vi "Channels Quiz - High Speed Streams and Tags.vi"() -> ()   [LabVIEW 2019]
doc: "After you have studied the other shipping examples to learn about channels, try this quiz to test your understanding."
uses:
  <extravilib>/ChannelInstances/High Speed Stream-i32/_Read For Replicate.vi
  <extravilib>/ChannelInstances/Tag-i32/Read With Abort.vi
  <extravilib>/ChannelInstances/Tag-i32/Write With Abort.vi
  <extravilib>/ChannelInstances/High Speed Stream-i32/Instantiate.vi
  <extravilib>/ChannelInstances/High Speed Stream-i32/)Channel.vi
  <extravilib>/ChannelInstances/High Speed Stream-i32/Abort Signal/Init Signal.vi
  <extravilib>/ChannelInstances/Tag-i32/Instantiate.vi
  <extravilib>/ChannelInstances/Tag-i32/EndpointRead.vi
  <extravilib>/ChannelInstances/Tag-i32/Endpoint.vi
  <extravilib>/ChannelInstances/High Speed Stream-i32.lvlib
  <extravilib>/ChannelInstances/Tag-i32.lvlib
panel:
  in  "Channel Type":string(combo)="High Speed Stream"
  out "element 1":i32
  in  "Stop Tag":bool
  in  "Stop Stream":bool
  out "element 0":i32
  # "Overview: Provides quiz questions related to several Channels concepts. You may wish to study the other channel examples first before attempting this quiz.\nInstructions:\n1. View the block diagram to see quiz questions related to High Speed Stream and Tag channel types.\n2. If you wish to run the VI to further understand the quiz answers, make sure you have specified the Channel Type that executes the diagram you wish to explore, and use the proper Stop button below to stop the VI."
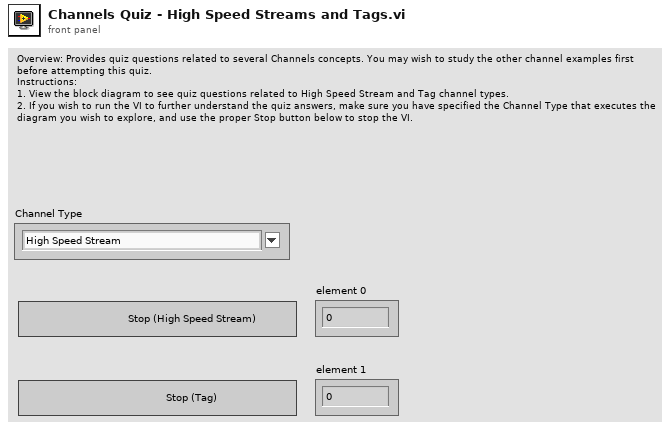
[diagram p1: front panel]
types:
  T1 = typedef "High Speed Stream-i32.lvlib/)Channel.ctl" = refnum<queue>
  T2 = typedef "Tag-i32.lvlib/))Channel.ctl" = refnum<queue>
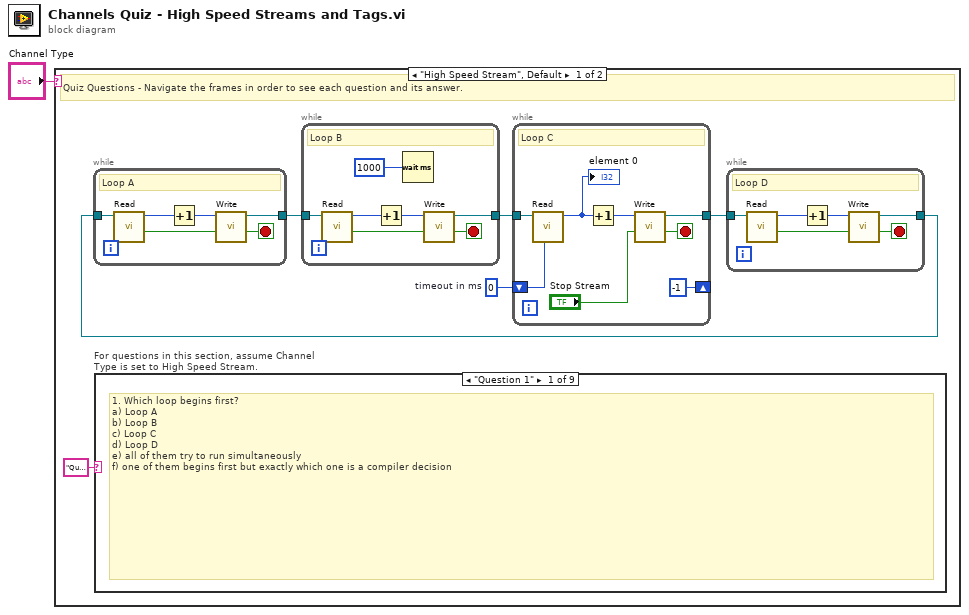
[diagram p0: block diagram]
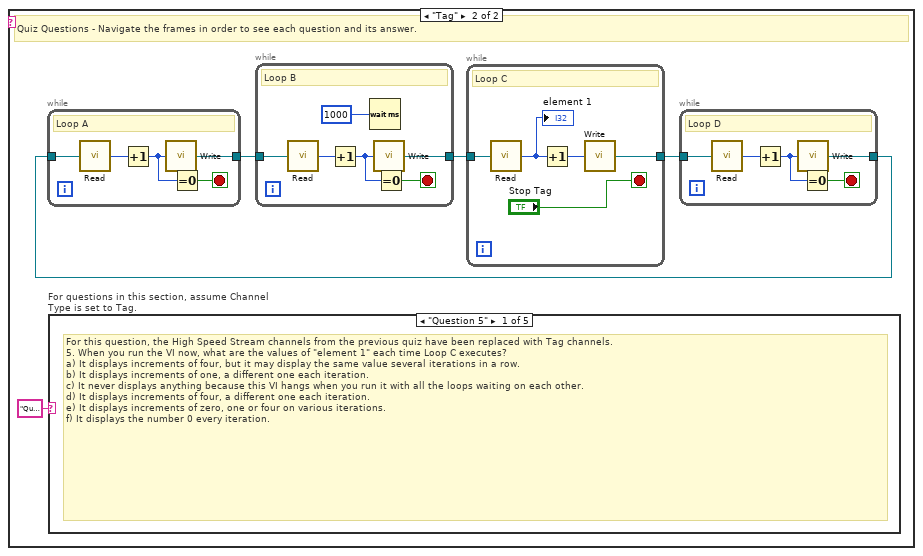
[diagram p10: hidden frame]
diagram:
  n1 = case shown="\"High Speed Stream\", Default" "Channel Type" {
    frame "High Speed Stream", Default {
      w3 = 0  # timeout in ms
      # "Quiz Questions - Navigate the frames in order to see each question and its answer."
      n2 = case "For questions in this section, assume Channel Type is set to High Speed Stream." shown="\"Question 1\"" "Question 1" {
        frame "Question 1" {
          # "1. Which loop begins first?\na) Loop A\nb) Loop B\nc) Loop C\nd) Loop D\ne) all of them try to run simultaneously\nf) one of them begins first but exactly which one is a compiler decision"
        }
        frame "Answer 1" {
          # "1. Which loop begins first?\na) Loop A\nb) Loop B\nc) Loop C\nd) Loop D\ne) all of them try to run simultaneously\nf) one of them begins first but exactly which one is a compiler decision\n\nAnswer: E. All try to begin at the same time. Channel wires do not create a dataflow dependency between the loops, so this is no different than four parallel while loops on a diagram. If you have enough CPU cores, LabVIEW will truly execute them in parallel."
        }
        frame "Question 2" {
          # "2. What are the values of \"element 0\" each time Loop C executes?\na) It displays increments of four, but it may display the same value several iterations in a row.\nb) It displays increments of one, a different one each iteration.\nc) It never displays anything because this VI hangs when you run it with all the loops waiting on each other.\nd) It displays increments of four, a different one each iteration.\ne) It displays increments of one most times but every once in a while the value increments by four in one iteration.\nf) It displays the number 0 every iteration."
        }
        frame "Answer 2" {
          # "2. What are the values of \"element 0\" each time Loop C executes?\na) It displays increments of four, but it may display the same value several iterations in a row.\nb) It displays increments of one, a different one each iteration.\nc) It never displays anything because this VI hangs when you run it with all the loops waiting on each other.\nd) It displays increments of four, a different one each iteration.\ne) It displays increments of one most times but every once in a while the value increments by four in one iteration.\nf) It displays the number 0 every iteration.\n\nAnswer: D. First value is zero. The zero is passed through the queues around the circle, getting incremented each time. When it comes back around, it is now 4. Repeat."
        }
        frame "Question 3" {
          # "3. If you deleted the Wait (ms) function from Loop C, what are the values of \"element 0\" each time the third loop executes?\na) It displays increments of four, but it may display the same value several iterations in a row.\nb) It displays increments of one, a different one each iteration.\nc) It never displays anything because this VI hangs when you run it with all the loops waiting on each other.\nd) It displays increments of four, a different one each iteration.\ne) It displays increments of one for the first two iterations but then starts incrementing by four each iteration.\nf) It displays the number 0 every iteration."
        }
        frame "Answer 3" {
          # "3. If you deleted the Wait (ms) function from Loop C, what are the values of \"element 0\" each time the third loop executes?\na) It displays increments of four, but it may display the same value several iterations in a row.\nb) It displays increments of one, a different one each iteration.\nc) It never displays anything because this VI hangs when you run it with all the loops waiting on each other.\nd) It displays increments of four, a different one each iteration.\ne) It displays increments of one for the first two iterations but then starts incrementing by four each iteration.\nf) It displays the number 0 every iteration.\n\nAnswer: D. No change in behavior. The same thing happens but faster."
        }
        frame "Question 4" {
          # "4. What happens when the Stop Stream button is pressed?\na) Nothing because the VI is hung with all loops waiting on each other.\nb) Loop C stops and the others keep running.\nc) Loop C stops and then the others stop in sequence so the VI halts.\nd) Loop D stops and then the others stop in sequence so that the VI halts.\ne) The loops stop iterating but the VI doesn't halt because the loops are waiting on each other to complete.\nf) The VI restarts as if the user had hit Abort and then hit the Run button again."
        }
        frame "Answer 4" {
          # "4. What happens when the Stop button is pressed?\na) Nothing because the VI is hung with all loops waiting on each other.\nb) Loop C stops and the others keep running.\nc) Loop C stops and then the others stop in sequence so the VI halts.\nd) Loop D stops and then the others stop in sequence so that the VI halts.\ne) The loops stop iterating but the VI doesn't halt because the loops are waiting on each other to complete.\nf) The VI restarts as if the user had hit Abort and then hit the Run button again.\n\nAnswer: C. The stop signal is propagated through this particular channel wire."
        }
        frame Default {
          # "End of Section 1. Please continue with the Tag case."
        }
      }
      n3 = while {
        tunnel: [w9] -> w7
        tunnel: w6 -> [w8]
        stop <- w10 stop-if-true
        # "Loop A"
        n4 = call <extravilib>:"Read.vi"("channel"=w8) -> ("done?"=w11:bool, "element"=w12:i32)  [unwired: 6 in, 3 out]
        n5 = Increment(x=w12) -> (x+1=w13:i32)
        n6 = call <extravilib>:"Write.vi"("last element? (F)"=w11, "element"=w13) -> ("done?"=w10:bool, "channel"=w9:T1)  [unwired: 7 in, 1 out]
      }
      n7 = while {
        tunnel: w7 -> [w16]
        tunnel: [w15] -> w5
        stop <- w17 stop-if-true
        # "Loop B"
        n8 = call <extravilib>:"Read.vi"("channel"=w16) -> ("done?"=w18:bool, "element"=w19:i32)  [unwired: 6 in, 3 out]
        n9 = Increment(x=w19) -> (x+1=w20:i32)
        n10 = Wait (ms)(milliseconds to wait=u32 1000) -> ()  [unwired: 1 out]
        n11 = call <extravilib>:"Write.vi"("last element? (F)"=w18, "element"=w20) -> ("done?"=w17:bool, "channel"=w15:T1)  [unwired: 7 in, 1 out]
      }
      n12 = while {
        tunnel: w5 -> [w25]
        tunnel: [w24] -> w4
        shift-right: [-1 ("timeout in ms")] -> _
        shift-left: w3 -> [w23]
        stop <- w26 stop-if-true
        # "Loop C"
        n13 = call <extravilib>:"Read.vi"("timeout in ms (-1)"=w23, "channel"=w25) -> ("element"=w27:i32)  [unwired: 5 in, 4 out]
        "element 0" <- w27
        n14 = Increment(x=w27) -> (x+1=w28:i32)
        n15 = call <extravilib>:"Write.vi"("last element? (F)"="Stop Stream", "element"=w28) -> ("done?"=w26:bool, "channel"=w24:T1)  [unwired: 7 in, 1 out]
      }
      n16 = while {
        tunnel: [w30] -> w6
        tunnel: w4 -> [w29]
        stop <- w31 stop-if-true
        # "Loop D"
        n17 = call <extravilib>:"Read.vi"("channel"=w29) -> ("done?"=w32:bool, "element"=w33:i32)  [unwired: 6 in, 3 out]
        n18 = Increment(x=w33) -> (x+1=w34:i32)
        n19 = call <extravilib>:"Write.vi"("last element? (F)"=w32, "element"=w34) -> ("done?"=w31:bool, "channel"=w30:T1)  [unwired: 7 in, 1 out]
      }
    }
    frame "Tag" {
      # "Quiz Questions - Navigate the frames in order to see each question and its answer."
      n20 = case "For questions in this section, assume Channel Type is set to Tag." shown="\"Question 5\"" "Question 5" {
        frame "Question 5" {
          # "For this question, the High Speed Stream channels from the previous quiz have been replaced with Tag channels.\n5. When you run the VI now, what are the values of \"element 1\" each time Loop C executes?\na) It displays increments of four, but it may display the same value several iterations in a row.\nb) It displays increments of one, a different one each iteration.\nc) It never displays anything because this VI hangs when you run it with all the loops waiting on each other.\nd) It displays increments of four, a different one each iteration.\ne) It displays increments of zero, one or four on various iterations.\nf) It displays the number 0 every iteration."
        }
        frame "Answer 5" {
          # "For this question, the High Speed Stream channels from the previous quiz have been replaced with Tag channels.\n5. When you run the VI, what are the values of \"element 1\" each time the third loop executes?\na) It displays increments of four, but it may display the same value several iterations in a row.\nb) It displays increments of one, a different one each iteration.\nc) It never displays anything because this VI hangs when you run it with all the loops waiting on each other.\nd) It displays increments of four, a different one each iteration.\ne) It displays increments of zero, one or four on various iterations.\nf) It displays the number 0 every iteration.\n\nAnswer: E. At the start, there are a couple of increment-by-one iterations. After that, the increment is either zero or four, depending upon whether Loop B has provided a new value or not."
        }
        frame "Question 6" {
          # "6. What happens when the Stop Tag button is pressed?\na) Nothing because the VI is hung with all loops waiting on each other.\nb) Loop C stops and the others keep running.\nc) Loop C stops and then the others stop in sequence so the VI halts.\nd) Loop D stops and then the others stop in sequence so that the VI halts.\ne) The loops stop iterating but the VI doesn't halt because the loops are waiting on each other to complete.\nf) The VI restarts as if the user had hit Abort and then hit the Run button again."
        }
        frame "Answer 6" {
          # "6. What happens when the Stop Tag button is pressed?\na) Nothing because the VI is hung with all loops waiting on each other.\nb) Loop C stops and the others keep running.\nc) Loop C stops and then the others stop in sequence so the VI halts.\nd) Loop D stops and then the others stop in sequence so that the VI halts.\ne) The loops stop iterating but the VI doesn't halt because the loops are waiting on each other to complete.\nf) The VI restarts as if the user had hit Abort and then hit the Run button again.\n\nAnswer: B. The signal to stop is not being propagated through the channels, so the other loops have no idea that they should stop. The value -1 never occurs, so the value +1 is never zero."
        }
        frame Default {
          # "End of Quiz"
        }
      }
      n21 = while {
        tunnel: [w43] -> w39
        tunnel: w38 -> [w42]
        stop <- w41 stop-if-true
        # "Loop A"
        n22 = call <extravilib>:"Read.vi"("channel"=w42) -> ("element"=w44:i32)  [unwired: 1 in, 1 out]
        n23 = Increment(x=w44) -> (x+1=w40:i32)
        n24 = call <extravilib>:"Write.vi"("element"=w40) -> ("channel"=w43:T2)  [unwired: 1 out]
        n25 = Equal To 0?(x=w40) -> (x = 0?=w41:bool)
      }
      n26 = while {
        tunnel: w39 -> [w49]
        tunnel: [w48] -> w37
        stop <- w46 stop-if-true
        # "Loop B"
        n27 = call <extravilib>:"Read.vi"("channel"=w49) -> ("element"=w50:i32)  [unwired: 1 in, 1 out]
        n28 = Increment(x=w50) -> (x+1=w45:i32)
        n29 = Wait (ms)(milliseconds to wait=u32 1000) -> ()  [unwired: 1 out]
        n30 = call <extravilib>:"Write.vi"("element"=w45) -> ("channel"=w48:T2)  [unwired: 1 out]
        n31 = Equal To 0?(x=w45) -> (x = 0?=w46:bool)
      }
      n32 = while {
        tunnel: w37 -> [w53]
        tunnel: [w52] -> w36
        stop <- "Stop Tag" stop-if-true
        # "Loop C"
        n33 = call <extravilib>:"Read.vi"("channel"=w53) -> ("element"=w54:i32)  [unwired: 1 in, 1 out]
        "element 1" <- w54
        n34 = Increment(x=w54) -> (x+1=w55:i32)
        n35 = call <extravilib>:"Write.vi"("element"=w55) -> ("channel"=w52:T2)  [unwired: 1 out]
      }
      n36 = while {
        tunnel: [w59] -> w38
        tunnel: w36 -> [w58]
        stop <- w57 stop-if-true
        # "Loop D"
        n37 = call <extravilib>:"Read.vi"("channel"=w58) -> ("element"=w60:i32)  [unwired: 1 in, 1 out]
        n38 = Increment(x=w60) -> (x+1=w56:i32)
        n39 = call <extravilib>:"Write.vi"("element"=w56) -> ("channel"=w59:T2)  [unwired: 1 out]
        n40 = Equal To 0?(x=w56) -> (x = 0?=w57:bool)
      }
    }
  }
